vi "创建运算类实例.vi"(8 "error in (no error)":errorcluster caption="错误输入（无错误）", 10 "运算":T1, 11 "运算工厂 输入":refnum<class "运算工厂.lvclass"> caption="DNL_LabVIEW Object in") -> (0 "error out":errorcluster caption="错误输出", 2 "运算类.lvclass":refnum<class "运算类.lvclass">, 3 "运算工厂 输出":refnum<class "运算工厂.lvclass"> caption="DNL_LabVIEW Object out")   [LabVIEW 2013, in "运算工厂.lvclass"]
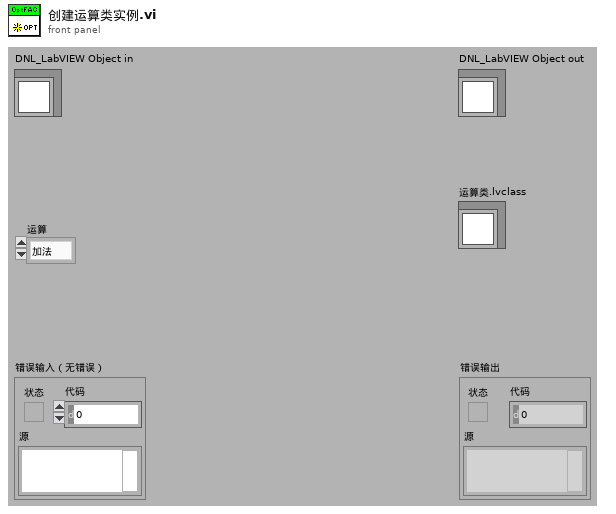
[diagram p1: front panel]
types:
  T1 = typedef "运算工厂.lvclass/运算方法.ctl" = enum16{"加法", "减法", "乘法", "平方和"}
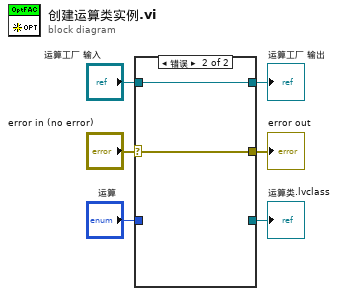
[diagram p0: block diagram]
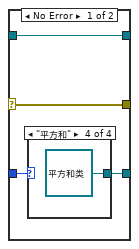
[diagram p2: hidden frame]
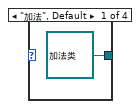
[diagram p3: hidden frame]
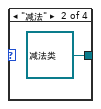
[diagram p4: hidden frame]
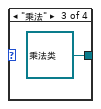
[diagram p5: hidden frame]
diagram:
  n1 = case shown="错误" "error in (no error)" {
    selector: "error in (no error)" -> [w9 w16]
    tunnel: [w9 w16] -> w5
    tunnel: [w10 w15] -> w3
    tunnel: "运算工厂 输入" -> [w10 w15]
    tunnel: "运算" -> [w8 _]
    tunnel: [w7 _] -> w1
    frame No Error {
      n2 = case shown="\"平方和\"" w8 {
        tunnel: [refnum<class "加法类.lvclass"> refnum ("加法类.lvclass") refnum<class "减法类.lvclass"> refnum ("减法类.lvclass") refnum<class "乘法类.lvclass"> refnum ("乘法类.lvclass") refnum<class "平方和类.lvclass"> refnum ("平方和类.lvclass")] -> w7
        frame "加法", Default {
        }
        frame "减法" {
        }
        frame "乘法" {
        }
        frame "平方和" {
        }
      }
    }
    frame Error {
    }
  }
  "error out" <- w5
  "运算工厂 输出" <- w3
  "运算类.lvclass" <- w1
